vi "test_exit.vi"() -> ()   [LabVIEW 2023]
uses:
  SECoP.lvlib
panel:
  in  "DLL path":path=path "D:/git-repos/shall-labview/64bit"
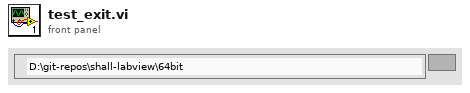
[diagram p1: front panel]
types:
  T1 = typedef "SECoP.lvlib/SECoP-libraries.ctl" = cluster{"serverDLL":path, "variantDLL":path, "cleanup_mode":bool, "Context_ID":string}
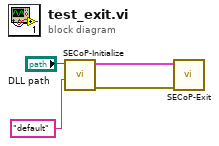
[diagram p0: block diagram]
diagram:
  n1 = call "SECoP-Initialize.vi"("Context ID (in)"="default", "DLL path (in)"="DLL path") -> ("error out"=w1:errorcluster, "DLL path (out)"=w2:T1)  [unwired: 8 in]
  n2 = call "SECoP-Exit.vi"("error in (no error)"=w1, "DLL path (in)"=w2) -> ()  [unwired: 9 in, 1 out]
